vi "Fct_calcul_vitesse_vent.vi"(11 "data":u32) -> (3 "Vent":dbl)   [LabVIEW 2017]
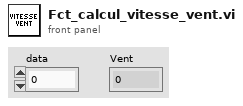
[diagram p1: front panel]
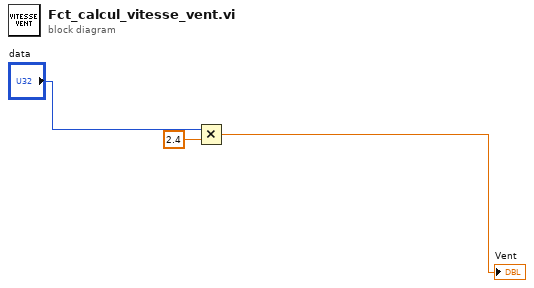
[diagram p0: block diagram]
diagram:
  n1 = Multiply(x="data", y=2.4) -> (x*y=→"Vent":dbl)
